vi "Client PC - Test Inbound Traffic to Server.vi"(8 "error in (no error)":errorcluster, 11 "ports to check":u16[](array[numeric])=[82, 482, 5672, 6343, 8002, 49580, 22, 44516, 52725, 8080]) -> (0 "error out":errorcluster, 2 "log file path":path, 3 "Results":string[][](array[string]))   [LabVIEW 2019]
doc: "Demonstrates how to set up a basic TCP connection, send data to the specified port once a connection has been established, and terminate the connection once the data has been sent. This VI is designed to stop if the TCP connection is terminated. The data sent in this example is an array of random numbers."
panel:
  out "log file name":string
  out "current test":cluster{string, "error out":errorcluster}
  in  "Start test":bool
  out "current port":u16
  out "Waveform Graph":dbl[](graph)
  # "1. Run the executable\n2. Open and run the Test Server Outboun Client PC on the client computer and follow the instructions on its front panel. Note that if you wait longer than 60 seconds to do this after running this VI, it will time out.\n3. Click on the button Start Test\n4. Click Stop to stop the VI. Note that if you stop the client VI, this VI will stop automatically."
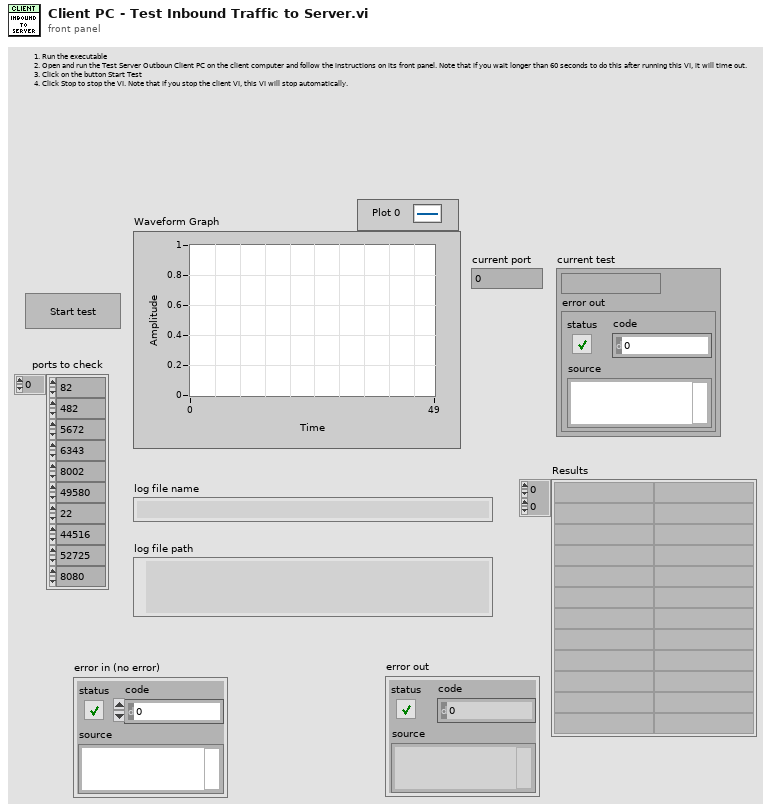
[diagram p1: front panel]
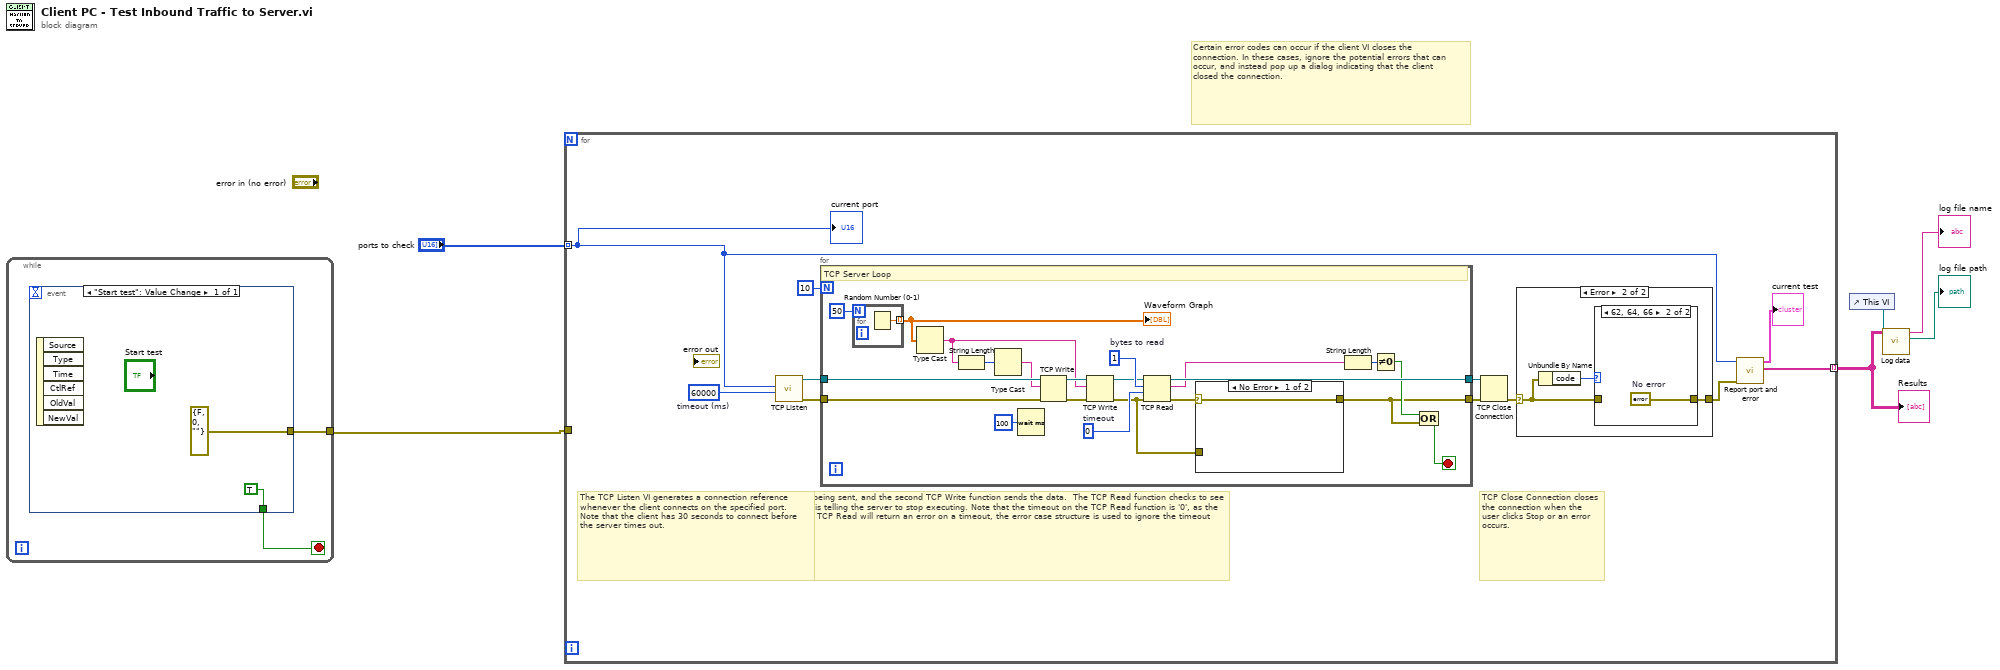
[diagram p0: block diagram]
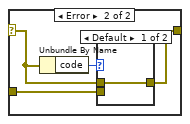
[diagram p2: hidden frame]
diagram:
  # "Certain error codes can occur if the client VI closes the connection. In these cases, ignore the potential errors that can occur, and instead pop up a dialog indicating that the client closed the connection."
  n1 = while {
    tunnel: [w8] -> w6
    stop <- w7 stop-if-true
    n2 = event shown="[0] \"Start test\": Value Change" {
      selector: _ -> [_]
      dyn-events: _ -> [_]
      timeout: _ -> [_]
      tunnel: [errorcluster {"status"=FALSE, "code"=0, "source"=""} ("error constant")] -> w8
      tunnel: [TRUE] -> w7
      event "Start test": Value Change {
        n3 = event-data() -> ()  [unwired: 1 in, 6 out]
      }
    }
  }
  n4 = for {
    tunnel: "ports to check" -> [w15] mode=indexing
    tunnel: w6 -> [_]
    tunnel: [w12] -> w5 mode=indexing
    w16 = 60000  # timeout (ms)
    # "TCP Close Connection closes the connection when the user clicks Stop or an error occurs."
    # "The TCP Listen VI generates a connection reference whenever the client connects on the specified port. Note that the client has 30 seconds to connect before the server times out."
    # "The first TCP Write function specifies the amount of data being sent, and the second TCP Write function sends the data.  The TCP Read function checks to see if the client has written any data. If it has, then the client is telling the server to stop executing. Note that the timeout on the TCP Read function is '0', as the client will not always be sending data to the server. Since TCP Read will return an error on a timeout, the error case structure is used to ignore the timeout error within the loop."
    n5 = call <vilib>:"TCP Listen.vi"("timeout ms (wait forever: -1)"=w16, "port"=w15) -> ("error out"=w17:errorcluster, "connection ID"=w18:refnum<k5>)  [unwired: 5 in, 3 out]
    n6 = for {
      N: 10 -> [_]
      tunnel: [w24] -> w20
      tunnel: [w30] -> w21
      tunnel: w18 -> [w42]
      tunnel: w17 -> [w34]
      stop <- w22 stop-if-true
      w29 = 0  # timeout
      w32 = 1  # bytes to read
      # "TCP Server Loop"
      n7 = for {
        N: 50 ("# of Points") -> [_]
        tunnel: [w50] -> w33 mode=indexing
        n8 = Random Number (0-1)() -> (number: 0 to 1=w50:dbl)
      }
      "Waveform Graph" <- w33
      n9 = Type Cast(x=w33) -> (*(type *) &x=w37:string)  [unwired: 1 out]
      n10 = String Length(string=w37) -> (length=w39:i32)
      n11 = Type Cast(x=w39) -> (*(type *) &x=w38:string)  [unwired: 1 out]
      n12 = Wait (ms)(milliseconds to wait=u32 100) -> ()  [unwired: 1 out]
      n13 = TCP Write(connection ID=w42, data in=w38, error in (no error)=w34) -> (connection ID out=w41:refnum<k5>, error out=w40:errorcluster)  [unwired: 2 out]
      n14 = TCP Write(connection ID=w41, data in=w37, error in (no error)=w40) -> (connection ID out=w31:refnum<k5>, error out=w23:errorcluster)  [unwired: 2 out]
      n15 = TCP Read(connection ID=w31, bytes to read=w32, error in (no error)=w23, 9:w29) -> (connection ID out=w30:refnum<k5>, data out=w27:string, error out=w25:errorcluster)  [unwired: 1 out]
      n16 = case shown="No Error" w25 {
        selector: w25 -> [w43 w46]
        tunnel: [w43 w44] -> w24
        tunnel: w23 -> [_ w45]
        frame No Error {
        }
        frame Error {
          n17 = Unbundle By Name(w46) -> ("code"=w47:i32)
          n18 = case shown="Default" w47 {
            tunnel: w46 -> [w48 _]
            tunnel: w45 -> [_ w49]
            tunnel: [w48 w49] -> w44
            frame Default {
            }
            frame 56 {
            }
          }
        }
      }
      n19 = String Length(string=w27) -> (length=w28:i32)
      n20 = Not Equal To 0?(x=w28) -> (x != 0?=w26:bool)
      n21 = Compound Arithmetic op=OR(w26, w24) -> (w22:bool)
    }
    n22 = TCP Close Connection(connection ID=w21, error in (no error)=w20) -> (error out=w19:errorcluster)  [unwired: 2 out]
    n23 = case shown="Error" w19 {
      selector: w19 -> [w51 w53]
      tunnel: [w51 w52] -> w14
      frame No Error {
      }
      frame Error {
        n24 = Unbundle By Name(w53) -> ("code"=w54:i32)
        n25 = case shown="62, 64, 66" w54 {
          tunnel: w53 -> [w55 _]
          tunnel: [w55 w56] -> w52
          frame Default {
          }
          frame 62, 64, 66 {
            w56 = errorcluster {"status"=FALSE, "code"=0, "source"=""}  # No error
          }
        }
      }
    }
    n26 = call "Report port and error.vi"("error in (no error)"=w14, "port"=w15) -> ("Array"=w12:string[], "output cluster"=→"current test":cluster{string, "error out":errorcluster})  [unwired: 7 in, 1 out]
    "current port" <- w15
  }
  "Results" <- w5
  n27 = control-ref of="This VI"() -> (w2:refnum<vi>)
  n28 = call "Log data.vi"(7:w2, 11:w5) -> ("log file path"=→"log file path":path, "log file name"=→"log file name":string)  [unwired: 7 in, 1 out]
